vi "Wavelet Edge Detection Helper.vi"(6 "Level":i32, 7 "Threshold ratio":dbl, 8 "error in (no error)":errorcluster, 9 "wavelet":u16, 10 "Image In":T1, 11 "Refnum in":T1) -> (0 "error out":errorcluster, 2 "Magnitude and Phase":cluster{dbl[][], dbl[][]}, 3 "Refnum out":T1)   [LabVIEW 2023]
uses:
  <vilib>/vision/Image Controls.llb/IMAQ Image.ctl
  <vilib>/addons/_Advanced Signal Processing/NI_AdvSigProcWA.lvlib
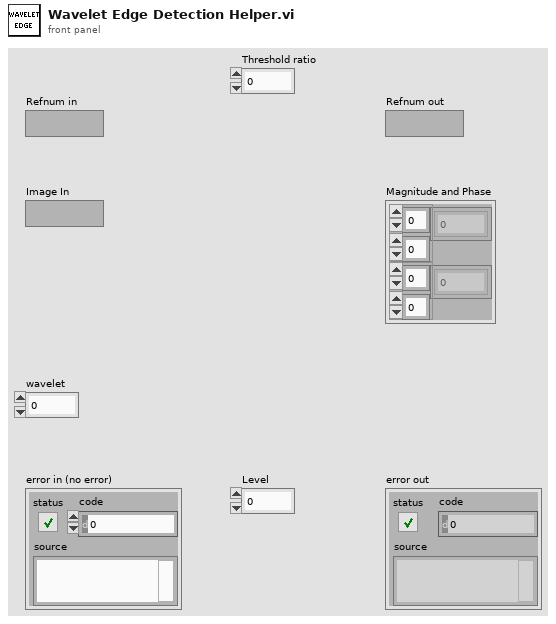
[diagram p1: front panel]
types:
  T1 = typedef "IMAQ Image.ctl" = refnum<image>
  T2 = typedef "Image Type" = u32
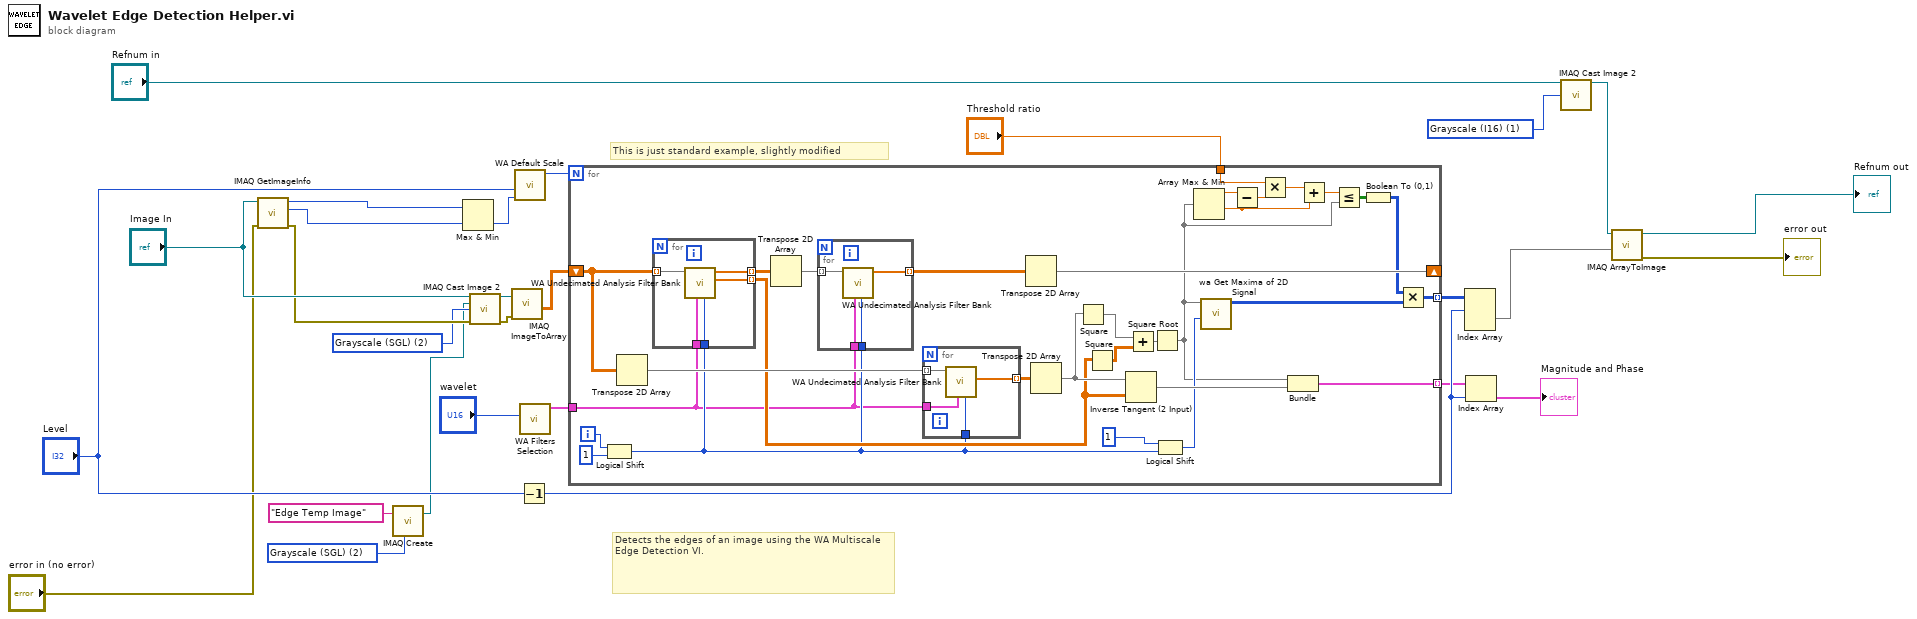
[diagram p0: block diagram]
diagram:
  w2 = T2 2 items=["Grayscale (U8)", "Grayscale (I16)", "Grayscale (SGL)", "Complex (CSG)", "RGB (U32)", "HSL (U32)", "RGB (U64)", "Grayscale (U16)"] ("Image Type")
  w6 = T2 1 items=["Grayscale (U8)", "Grayscale (I16)", "Grayscale (SGL)", "Complex (CSG)", "RGB (U32)", "HSL (U32)", "RGB (U64)", "Grayscale (U16)"] ("Image Type")
  w9 = T2 2 items=["Grayscale (U8)", "Grayscale (I16)", "Grayscale (SGL)", "Complex (CSG)", "RGB (U32)", "HSL (U32)", "RGB (U64)", "Grayscale (U16)"] ("Image Type")
  # "This is just standard example, slightly modified"
  # "Detects the edges of an image using the WA Multiscale Edge Detection VI."
  n1 = call "IMAQ GetImageInfo"("error in (no error)"="error in (no error)", "Image"="Image In") -> ("error out"=w11:errorcluster, "Y Resolution"=w13:i32, "X Resolution"=w14:i32)  [unwired: 2 in, 5 out]
  n2 = call "IMAQ Create"("Image Name"="Edge Temp Image", "Image Type"=w2) -> ("New Image"=w1:T1)  [unwired: 3 in, 1 out]
  n3 = Max & Min(x=w14, y=w13) -> (min(x,y)=w26:i32)  [unwired: 1 out]
  n4 = call "IMAQ Cast Image 2"("Image Src"="Image In", "Image Dst"=w1, "Image Type"=w9, "error in (no error)"=w11) -> ("Image Dst Out"=w10:T1, "error out"=w8:errorcluster)  [unwired: 10 in]
  n5 = call "IMAQ ImageToArray"("error in (no error)"=w8, "Image"=w10) -> ("Image Pixels (Float)"=w27:sgl[][])  [unwired: 2 in, 4 out]
  n6 = call <vilib>:"WA Default Scale.vi"("signal length"=w26, "level in"="Level") -> ("level out"=w17:i32)  [unwired: 1 in, 4 out]
  n7 = Decrement(x="Level") -> (x-1=w24:i32)
  n8 = call <vilib>:"WA Filters Selection.vi"("wavelet"="wavelet") -> ("analysis filters"=w18:cluster{"lowpass":dbl[], "highpass":dbl[]})  [unwired: 2 in, 8 out]
  n9 = for {
    N: w17 -> [_]
    shift-right: [w56] -> _
    shift-left: w27 -> [w53]
    tunnel: [w47] -> w23 mode=indexing
    tunnel: w18 -> [w39]
    tunnel: "Threshold ratio" -> [w32]
    tunnel: [w29] -> w21 mode=indexing
    i -> [w44]
    n10 = Logical Shift(y=w44, x=1) -> (x << y=w41:i32)
    n11 = Transpose 2D Array(2D array=w53) -> (transposed array=w55:dbl[][])
    n12 = for {
      tunnel: w53 -> [w72] mode=indexing
      tunnel: [w71] -> w45 mode=indexing
      tunnel: [w70] -> w59 mode=indexing
      tunnel: w41 -> [w69]
      tunnel: w39 -> [w68]
      n13 = call <vilib>:"WA Undecimated Analysis Filter Bank.vi"("factor"=w69, "analysis filters"=w68, "X"=w72) -> ("Detail Coeffs"=w71:dbl[], "Apprx Coeffs"=w70:dbl[])  [unwired: 2 in, 5 out]
    }
    n14 = Transpose 2D Array(2D array=w59) -> (transposed array=w58:dbl[][])
    n15 = for {
      tunnel: w58 -> [w67] mode=indexing
      tunnel: [w66] -> w57 mode=indexing
      tunnel: w41 -> [w65]
      tunnel: w39 -> [w64]
      n16 = call <vilib>:"WA Undecimated Analysis Filter Bank.vi"("factor"=w65, "analysis filters"=w64, "X"=w67) -> ("Apprx Coeffs"=w66:dbl[])  [unwired: 2 in, 6 out]
    }
    n17 = for {
      tunnel: w55 -> [w63] mode=indexing
      tunnel: [w62] -> w54 mode=indexing
      tunnel: w41 -> [w61]
      tunnel: w39 -> [w60]
      n18 = call <vilib>:"WA Undecimated Analysis Filter Bank.vi"("factor"=w61, "analysis filters"=w60, "X"=w63) -> ("Detail Coeffs"=w62:dbl[])  [unwired: 2 in, 6 out]
    }
    n19 = Transpose 2D Array(2D array=w57) -> (transposed array=w56:dbl[][])
    n20 = Transpose 2D Array(2D array=w54) -> (transposed array=w46:dbl[][])
    n21 = Square(x=w46) -> (x^2=w51:dbl[][])
    n22 = Square(x=w45) -> (x^2=w52:dbl[][])
    n23 = Inverse Tangent (2 Input)(1:w45, 2:w46) -> (0:w48:dbl[][])
    n24 = Add(x=w51, y=w52) -> (x+y=w50:dbl[][])
    n25 = Square Root(x=w50) -> (sqrt(x)=w31:dbl[][])
    n26 = Logical Shift(y=1, x=w41) -> (x << y=w42:i32)
    n27 = Array Max & Min(array=w31) -> (max value=w34:dbl, min value=w36:dbl)  [unwired: 2 out]
    n28 = call <vilib>:"wa Get Maxima of 2D Signal.vi"("range"=w42, "Image"=w31) -> ("Edge"=w49:i16[][])  [unwired: 9 out]
    n29 = Subtract(x=w34, y=w36) -> (x-y=w35:dbl)
    n30 = Multiply(x=w32, y=w35) -> (x*y=w37:dbl)
    n31 = Bundle(w31, w48) -> (w47:cluster{dbl[][], dbl[][]})  [unwired: 1 out]
    n32 = Add(x=w37, y=w36) -> (x+y=w38:dbl)
    n33 = Less Or Equal?(x=w38, y=w31) -> (x <= y?=w33:bool[][])
    n34 = Boolean To (0,1)(Boolean=w33) -> (0, 1=w30:i16[][])
    n35 = Multiply(x=w30, y=w49) -> (x*y=w29:i16[][])
  }
  n36 = Index Array(array=w21, index (dim 0)=w24) -> (element=w22:i16[][])  [unwired: 2 in]
  n37 = Index Array(array=w23, index=w24) -> (element=→"Magnitude and Phase":cluster{dbl[][], dbl[][]})
  n38 = call "IMAQ Cast Image 2"("Image Src"="Refnum in", "Image Type"=w6) -> ("Image Dst Out"=w4:T1)  [unwired: 12 in, 1 out]
  n39 = call "IMAQ ArrayToImage"("Image Pixels (I16)"=w22, "Image"=w4) -> ("error out"=→"error out":errorcluster, "Image Out"=→"Refnum out":T1)  [unwired: 8 in]
